vi "EEG_2022_040_LabView_3.4.vi"() -> ()   [LabVIEW 2022 SP3]
panel:
  out "Temperature History":ext(graph)
  in  "stop":bool
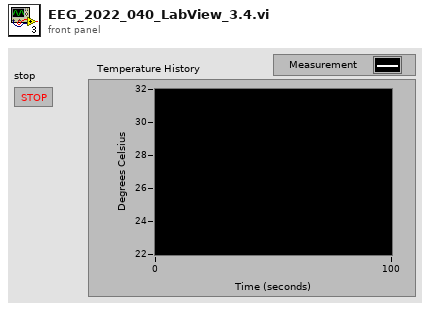
[diagram p1: front panel]
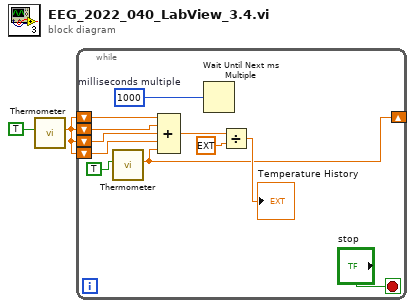
[diagram p0: block diagram]
diagram:
  n1 = call "Thermometer.vi"("Temp Scale"=TRUE) -> ("Temperature"=w2:dbl)  [unwired: 9 in, 1 out]
  n2 = while {
    shift-right: [w8] -> _
    shift-left: w2 -> [w4]
    shift-left: w2 -> [w5]
    shift-left: w2 -> [w6]
    shift-left: w2 -> [w7]
    stop <- "stop" stop-if-true
    w13 = 1000  # milliseconds multiple
    n3 = call "Thermometer.vi"("Temp Scale"=TRUE) -> ("Temperature"=w8:dbl)  [unwired: 9 in, 1 out]
    n4 = Compound Arithmetic op=ADD(w7, w6, w5, w4, w8) -> (w11:dbl)
    n5 = Wait Until Next ms Multiple(millisecond multiple=w13) -> ()  [unwired: 1 out]
    n6 = Divide(x=w11, y=ext 5.0) -> (x/y=→"Temperature History":ext)
  }
